vi "Keithley24xx_Meash_FE.vi"(0 "b_VISA In":refnum<visa-resource-name>, 1 "c_VISA In":refnum<visa-resource-name>, 2 "Ic,A":dbl, 5 "MeasF In":string, 7 "Step ,A":dbl, 9 "c_Err In":errorcluster, 11 "b_Err In":errorcluster, 12 "Begin Level Ibase, A":dbl, 13 "Ibase max,A":dbl) -> (4 "c_VISA Out":refnum<visa-resource-name>, 6 "b_VISA Out":refnum<visa-resource-name>, 8 "hFE":dbl format="%#.3g", 10 "c_Err Out":errorcluster, 15 "b_Err Out":errorcluster)   [LabVIEW 2014]
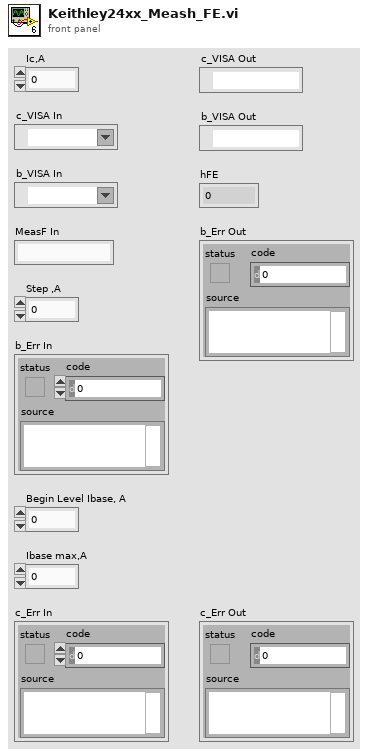
[diagram p1: front panel]
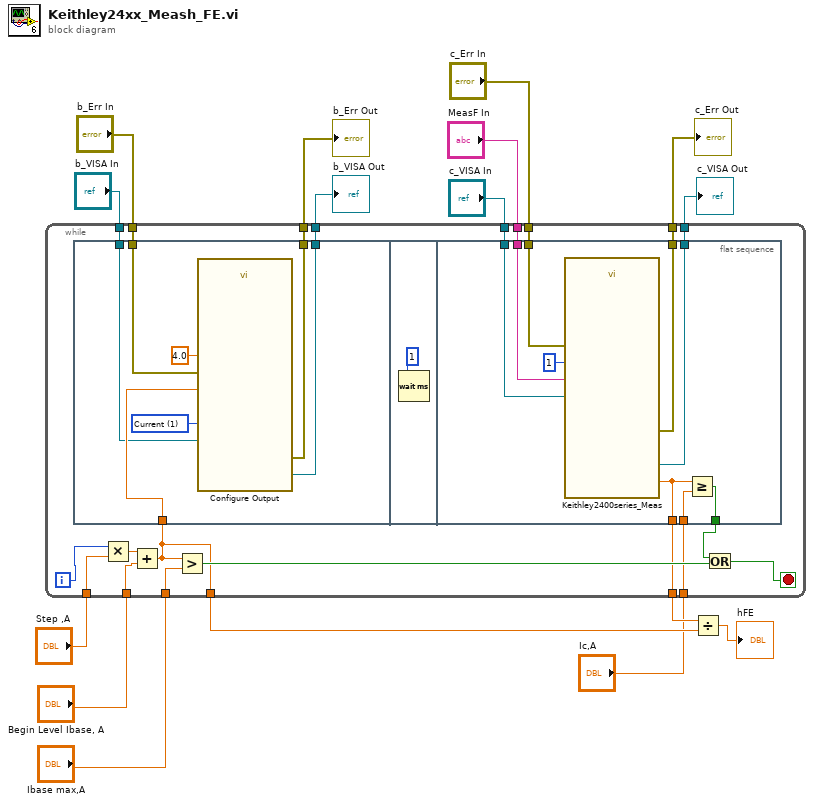
[diagram p0: block diagram]
diagram:
  n1 = while {
    tunnel: "Step ,A" -> [w31]
    tunnel: "Begin Level Ibase, A" -> [w30]
    tunnel: "Ibase max,A" -> [w29]
    tunnel: [w28] -> w15
    tunnel: [w27] -> w14
    tunnel: "MeasF In" -> [w26]
    tunnel: "c_VISA In" -> [w25]
    tunnel: "c_Err In" -> [w24]
    tunnel: "b_VISA In" -> [w23]
    tunnel: "b_Err In" -> [w22]
    tunnel: [w21] -> w5
    tunnel: [w20] -> w4
    tunnel: [w19] -> w3
    tunnel: [w18] -> w2
    tunnel: "Ic,A" -> [w17]
    i -> [w32]
    stop <- w33 stop-if-true
    n2 = flat-sequence {
      tunnel: w27 -> [w41]
      tunnel: w23 -> [w40]
      tunnel: w22 -> [w39]
      tunnel: [w38] -> w21
      tunnel: [w37] -> w20
      tunnel: [w52] -> w34
      tunnel: [w51] -> w28
      tunnel: w26 -> [w50]
      tunnel: w25 -> [w49]
      tunnel: w24 -> [w48]
      tunnel: [w47] -> w19
      tunnel: [w46] -> w18
      tunnel: w17 -> [w45]
      frame #0 {
        w43 = u16 1 items=["Voltage", "Current"] ("Source Mode  (0: Voltage)")
        n3 = call "Configure Output.vi"("Source Mode  (0: Voltage)"=w43, "error in (no error)"=w39, "Compliance  Level (0.1)"=4.0, "Output Level (0)"=w41, "VISA resource name"=w40) -> ("error out"=w38:errorcluster, "VISA resource name out"=w37:refnum<visa-resource-name>)  [unwired: 5 in]
      }
      frame #1 {
        n4 = Wait (ms)(milliseconds to wait=u32 1) -> ()  [unwired: 1 out]
      }
      frame #2 {
        n5 = call "Keithley2400series_Meas.vi"("MEAS:<f>"=w50, "error in (no error)"=w48, "MEAS mode, 0 Volt"=u16 1, "VISA resource name in"=w49) -> ("error out"=w47:errorcluster, "Замер"=w51:dbl, "VISA out"=w46:refnum<visa-resource-name>)  [unwired: 1 in, 1 out]
        n6 = Greater Or Equal?(x=w51, y=w45) -> (x >= y?=w52:bool)
      }
    }
    n7 = Multiply(x=w32, y=w31) -> (x*y=w36:dbl)
    n8 = Add(x=w36, y=w30) -> (x+y=w27:dbl)
    n9 = Greater?(x=w27, y=w29) -> (0:w35:bool)
    n10 = Or(x=w34, y=w35) -> (x .or. y?=w33:bool)
  }
  "c_VISA Out" <- w2
  "b_VISA Out" <- w4
  "b_Err Out" <- w5
  "c_Err Out" <- w3
  n11 = Divide(x=w15, y=w14) -> (x/y=→"hFE":dbl)
